vi "fill_zero_pre_numeric.vi"(0 "Numeric":u16, 1 "digit number":u8=3) -> (2 "concatenated string":string="000")   [LabVIEW 2020]
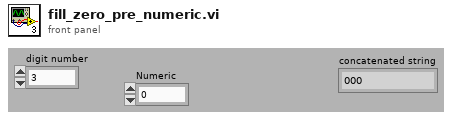
[diagram p1: front panel]
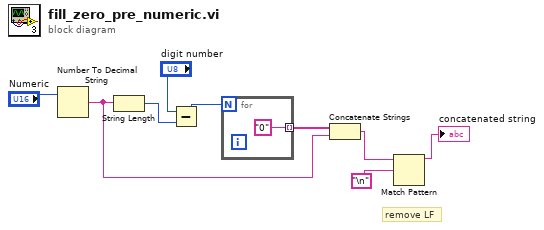
[diagram p0: block diagram]
diagram:
  # "remove LF"
  n1 = Number To Decimal String(number="Numeric") -> (decimal integer string=w4:string)  [unwired: 1 out]
  n2 = String Length(string=w4) -> (length=w7:i32)
  n3 = Subtract(x="digit number", y=w7) -> (x-y=w6:i32)
  n4 = for {
    N: w6 -> [_]
    tunnel: ["0"] -> w5 mode=indexing
  }
  n5 = Concatenate Strings(w5, w4) -> (w3:string)
  n6 = Match Pattern(string=w3, regular expression="\n") -> (before substring=→"concatenated string":string)  [unwired: 1 in, 3 out]
